vi "Update lookup table of devices on system.vi"(8 "error in (no error)":errorcluster, 10 "Hardware Resources":refnum<k20>[](array[refnum]) caption="Resources out", 11 "Controller in":refnum<class "Controller.lvclass">) -> (0 "error out":errorcluster, 3 "Controller out":refnum<class "Controller.lvclass">)   [LabVIEW 2026, in "Controller Actor.lvlib" / "Controller.lvclass"]
uses:
  Controller.lvclass
  Controller.lvclass/Controller.ctl
  <resource>/objmgr/nicontrollersysapi.rc
  <resource>/objmgr/pxisysapi.rc
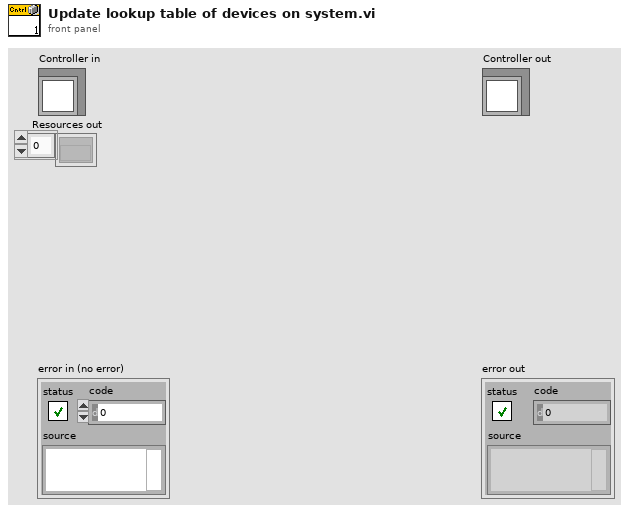
[diagram p1: front panel]
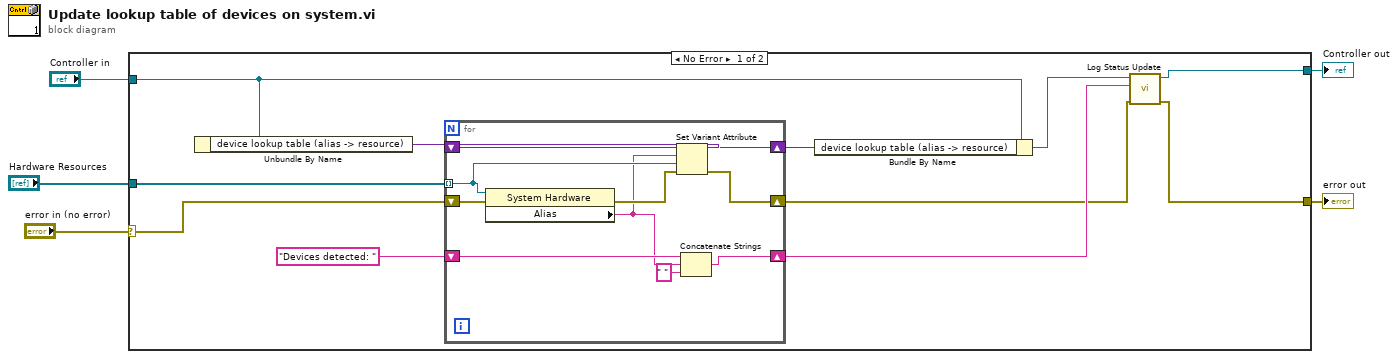
[diagram p0: block diagram]
diagram:
  n1 = case shown="No Error" "error in (no error)" {
    selector: "error in (no error)" -> [w16 w28]
    tunnel: [w6 w28] -> w4
    tunnel: [w10 w27] -> w2
    tunnel: "Controller in" -> [w15 w27]
    tunnel: "Hardware Resources" -> [w12 _]
    frame No Error {
      n2 = Unbundle By Name(w15) -> ("device lookup table (alias -> resource)"=w14:variant)
      n3 = for {
        shift-right: [w22] -> w7
        shift-left: w16 -> [w26]
        shift-right: [w23] -> w13
        shift-left: w14 -> [w24]
        tunnel: w12 -> [w21] mode=indexing
        shift-right: [w19] -> w8
        shift-left: "Devices detected: " -> [w20]
        n4 = property class="System Hardware"(reference=w21, error in=w26) -> (error out=w25:errorcluster, "Alias"=w18:string)  [unwired: 1 out]
        n5 = Set Variant Attribute(Variant=w24, name=w18, value=w21, error in=w25) -> (Variant out=w23:variant, error out=w22:errorcluster)  [unwired: 1 out]
        n6 = Concatenate Strings(w20, w18, " " ("string")) -> (w19:string)
      }
      n7 = Bundle By Name(cluster=w15, "device lookup table (alias -> resource)"=w13) -> (w11:refnum<class "Controller.lvclass">)
      n8 = call-dynamic "Log Status Update.vi"("error in (no error)"=w7, "String"=w8, "Controller in"=w11) -> ("error out"=w6:errorcluster, "Controller out"=w10:refnum<class "Controller.lvclass">)  [unwired: 7 in]
    }
    frame Error {
    }
  }
  "error out" <- w4
  "Controller out" <- w2
